vi "Logarithm of Complete Gamma Function.vi"(3 "x":dbl format="%.2f") -> (1 "ln(g(x))":dbl format="%.2f")   [LabVIEW 2017, in "NI_Gmath.lvlib"]
doc: "Computes the natural logarithm of the complete gamma function."
uses:
  NI_Gmath.lvlib
  lvanlys.dll
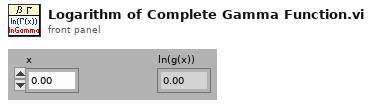
[diagram p1: front panel]
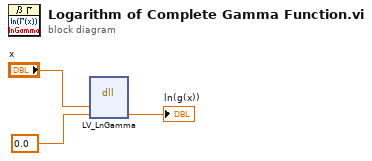
[diagram p0: block diagram]
diagram:
  n1 = dll-call lib="C:/Program Files/National Instruments/LabVIEW 2017/resource/lvanlys.*" fn="LV_LnGamma"("x"="x", "ln(Gamma(x))"=0.0 ("Gamma")) -> ("ln(Gamma(x))"=→"ln(g(x))":dbl)  [unwired: 5 in, 2 out]
